vi "data buffer.vi"(4 "Error In":errorcluster, 7 "Instance Name":T1) -> (0 "Error Out":errorcluster, 3 "DVR":refnum<data-value>)   [LabVIEW 2015, in "Temperature Controller Data Buffer.lvlib"]
uses:
  Temperature Controller Data Buffer.lvlib
  _libraries/Startup Processes/_typedefs/Subpanel Names.ctl
  buffer data typedef.ctl
  _libraries/Startup Processes/Startup Processes.lvlib
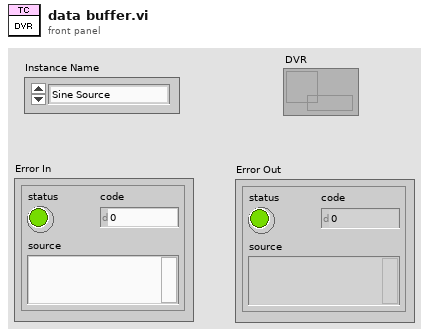
[diagram p1: front panel]
types:
  T1 = typedef "Startup Processes.lvlib/Subpanel Names.ctl" = enum16{"Sine Source", "Ramp Source", "Hen House TC", "Dog House TC", "Out House TC"}
  T2 = typedef "Temperature Controller Data Buffer.lvlib/buffer data typedef.ctl" = cluster{"TC Data":cluster{"Last value":dbl, "Error High Level":dbl, "Warning High Level":dbl, "Warning Low Level":dbl, "Error Low Level":dbl}[], "Counter":i32}
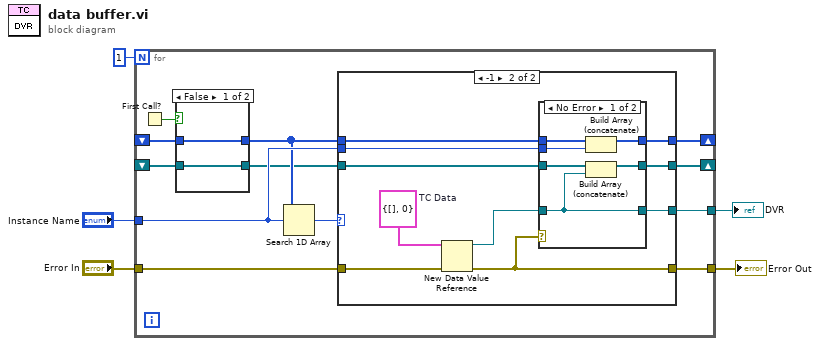
[diagram p0: block diagram]
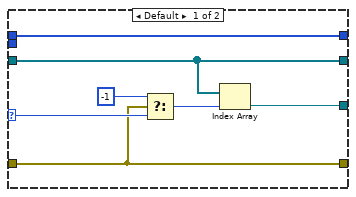
[diagram p3: hidden frame]
diagram:
  n1 = for {
    N: 1 -> [_]
    tunnel: "Error In" -> [w17]
    tunnel: [w16] -> w4
    shift-right: [w12] -> _
    shift-left: _ -> [w7]
    shift-right: [w14] -> _
    shift-left: _ -> [w10]
    tunnel: "Instance Name" -> [w13]
    tunnel: [w11] -> w1
    n2 = First Call?() -> (First Call?: T/F=w9:bool)
    n3 = case shown="False" w9 {
      tunnel: w7 -> [w18 _]
      tunnel: w10 -> [w19 _]
      tunnel: [w19 _] -> w8
      tunnel: [w18 _] -> w6
      frame False {
      }
      frame True {
      }
    }
    n4 = Search 1D Array(1D array=w8, element=w13) -> (index of element=w15:i32)  [unwired: 1 in]
    n5 = case shown="-1" w15 {
      selector: w15 -> [w22 _]
      tunnel: w17 -> [w21 w36]
      tunnel: [w21 w34] -> w16
      tunnel: [w26 w32] -> w14
      tunnel: w8 -> [w26 w33]
      tunnel: w13 -> [_ w31]
      tunnel: w6 -> [w24 w30]
      tunnel: [w24 w29] -> w12
      tunnel: [w25 w27] -> w11
      frame Default {
        n6 = Select(t=-1, s=w21, f=w22) -> (s? t:f=w23:i32)
        n7 = Index Array(array=w24, index=w23) -> (element=w25:refnum<data-value>)
      }
      frame -1 {
        w35 = T2 {"TC Data"=[], "Counter"=0}  # TC Data
        n8 = New Data Value Reference(data value=w35, error in=w36) -> (data value reference=w28:refnum<data-value>, error out=w34:errorcluster)
        n9 = case shown="No Error" w34 {
          tunnel: w33 -> [w42 w45]
          tunnel: [w40 w45] -> w32
          tunnel: w31 -> [w41 _]
          tunnel: w30 -> [w39 w44]
          tunnel: w28 -> [w37 w43]
          tunnel: [w38 w44] -> w29
          tunnel: [w37 w43] -> w27
          frame No Error {
            n10 = Build Array (concatenate)(w42, w41) -> (w40:T1[])
            n11 = Build Array (concatenate)(w39, w37) -> (w38:refnum<data-value>[])
          }
          frame Error {
          }
        }
      }
    }
  }
  "Error Out" <- w4
  "DVR" <- w1
